vi "3DViewEye.vi"(0 "Choose Directory":path) -> ()   [LabVIEW 2022 SP3]
uses:
  <vilib>/Analysis/NI_AALPro.lvlib
  <vilib>/Analysis/4window.llb/Chebyshev Window (DBL).vi
  <vilib>/Math Plots/3D Math Plots/3D Surface/3D Surface Datatype/3D Surface Datatype.lvclass
  <vilib>/Math Plots/3D Math Plots/3D Surface/3D Surface Datatype/Public/Plot Helper (Vector).vi
  <vilib>/Math Plots/3D Math Plots/3D Surface/3D Surface XCtrl/3D Surface.xctl
panel:
  in  "length":i32
  in  "index":i32
  out "3D Surface":refnum<class "3D Plot Datatype.lvclass">[](xcontrol)
  out "Peaks":dbl[](graph)
  in  "# rings":i32=1
  in  "Fix dB Range?":bool
  in  "Parse":u16=1
  in  "Filter Prams":T1={"low cutoff"=5, "order"=81, "high cutoff"=35}
  in  "Type of Mean":u16(ring)=3 items=["Mean from lines", "Mean just lines", "Poly Mean", "No mean", "Filter"]
  in  "Flip?":bool=TRUE
  in  "Compress":bool
  in  "Y scale":dbl=1.0
  in  "X scale":dbl=1.0
  in  "file ext":string="*.eye"
  out "Current Image":string
  out "Numeric":i32
  out "Array":dbl[](array[numeric])
  in  "Save Data":bool
  in  "Use Selected Files":bool
  in  "Listbox":i32[](listbox)
  out "Scale factors":dbl[](array[numeric])
  out "BMP to be":dbl[][](graph)
  # "Slect a batch of eye files and the will be saved as BMP 24 bit RGB. They will be converted to a 1to1 aspect ratio and the batch will be scaled to reflect absolute voltage levels. Data is log compressed. May want to adjust Z scale to improve contrast."
  # "Scale in mm"
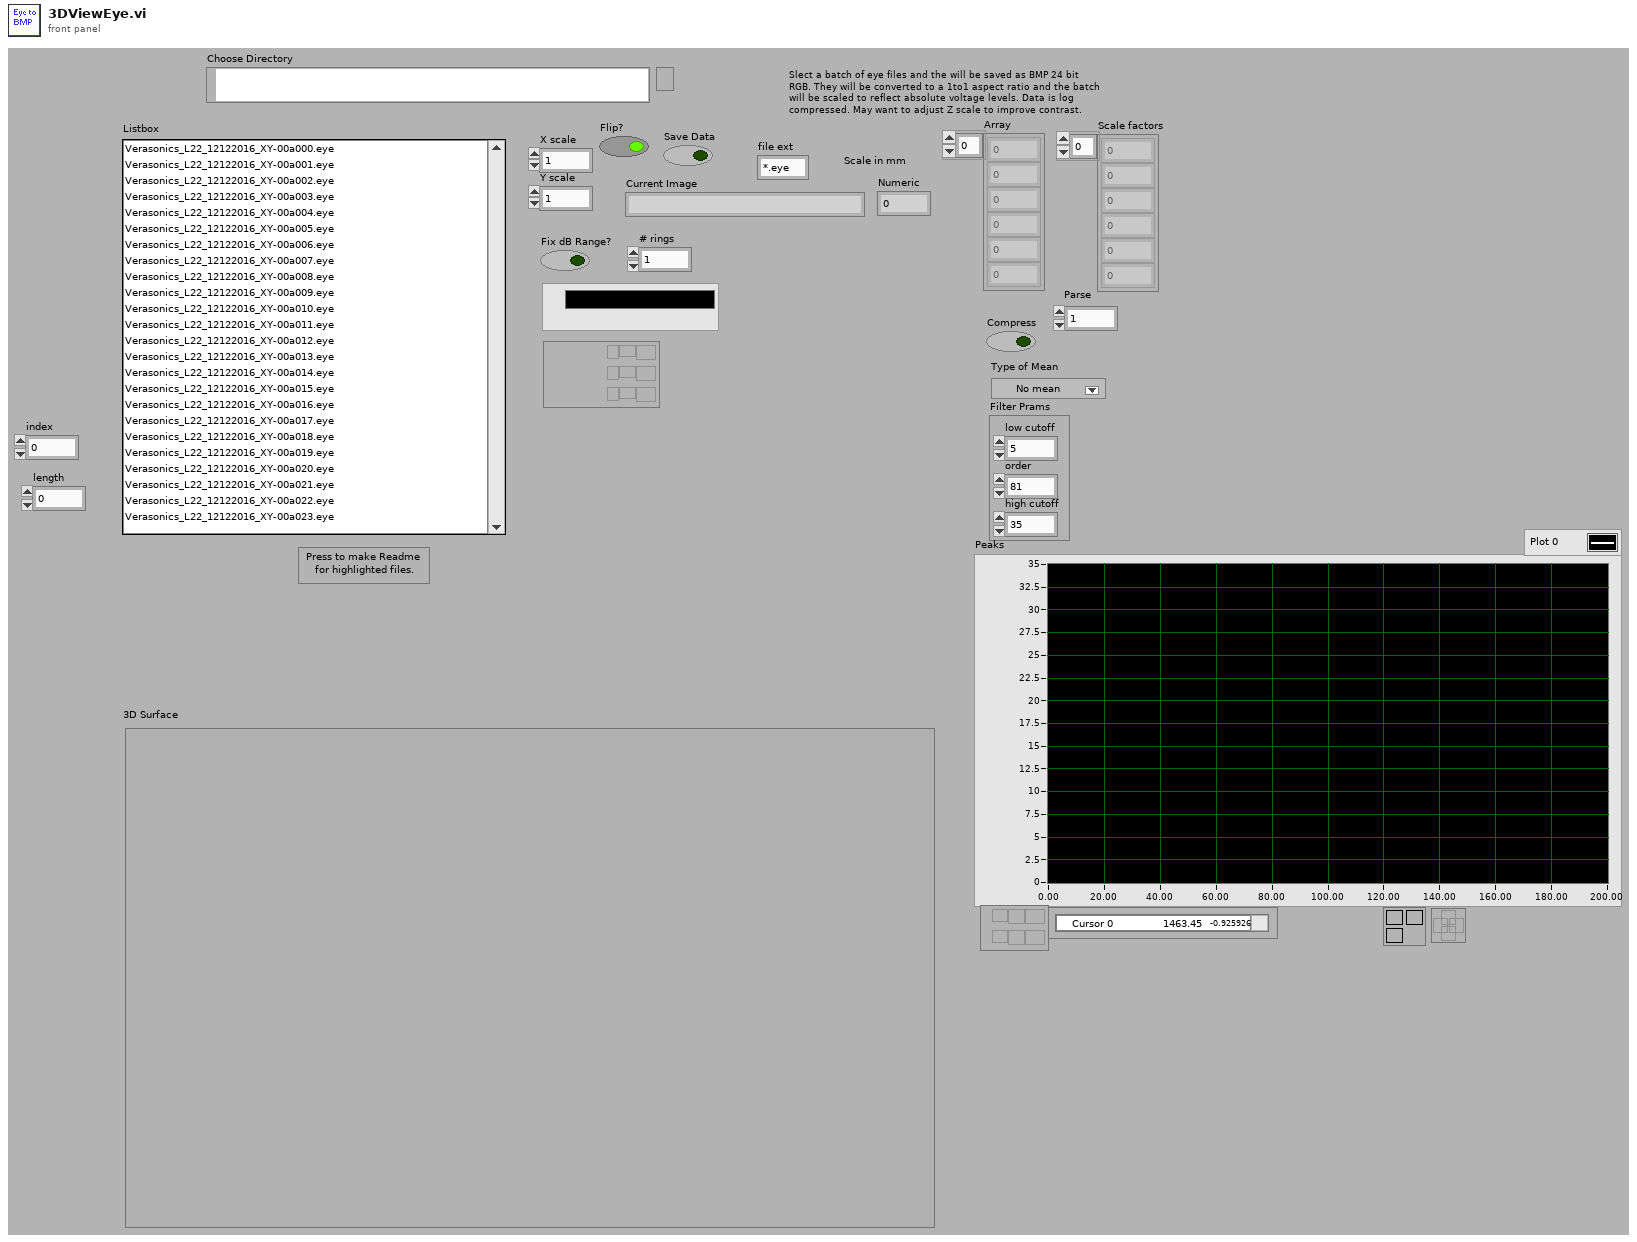
[diagram p1: front panel]
types:
  T1 = cluster{"low cutoff":i32, "order":i32, "high cutoff":i32}
  T2 = typedef "Header.ctl" = cluster{"header info":cluster{"Header":string, "Head length":i16}, "A/D info":cluster{"# rf points per line":u16, "# lines per scan":u16, "sample rate MHz":u16, "# A/D bits":i16, "# bytes per A/D":u16, "TGC Flag":u16, "A/D Type":string}, "Tranducer Info":cluster{"bandwidth":sgl, "center freq":sgl, "start freq":sgl, "ID":i32}, "Scan Info":cluster{"delay":sgl, "pivot distance":sgl, "sector scan angle":sgl, "operator":string, "Scan Mode":string, "location":string}, "Time/Date Info":cluster{"date":string, "time":string}, "RF Info":cluster{"RF file name":string, "RF file att":string, "RF cal file name":string, "RF cal file att":string}, "Patient Info":cluster{"ID":string, "extended ID":string, "age":u16, "sex":string, "previously\nscanned":string, "PSA":sgl, "LOS":u8, "Ethnicty 2":u8, "Race":u8}, "Tissue Type":cluster{"organ":i16, "disease type":i16, "disease location":i16, "IQ_pts":u16, "RcvBuffer":u8, "RcvFrame":u16, "IQBuff":u8, "IQFrame":u16, "IQPage":u8}, "Votage scaling":cluster{"Digitizer (dB)":sgl, "Gain (dB)":sgl, "Atten (dB)":sgl}, "Comment":string, "Misc Info":cluster{"avg num":u16, "c speed":i16, "Div By or SF zones":i16, "XMIT CHS":u8, "RCV CHS":u8, "Xmit angle":sgl}, "Therapy Parameters":cluster{"Theraputic Freq (MHz)":sgl, "Time on (s)":sgl, "Therapy amplitude (mV)":sgl, "Lines Before":u16, "Lines After":u16}, "Scan Settings":cluster{"Energy (uJ or V)":u8, "Damp (Ohm) or Fc":u8, "HP Filt (KHz)":u8, "LP Filt (MHz)":u8, "Gain (db)":u8, "prf (kHz)":sgl, "Distance between\nscan lines (um)":u16, "Distance between\nscan planes (um)":u16, "Scan line gap (um)":sgl, "Scan plane gap (um)":sgl}, "Compression Parameters":cluster{"F1 (MHz)":sgl, "F2 (MHz)":sgl, "% taper":sgl, "duration":sgl}, "Patient Info Xtra":cluster{"First Name":string, "Last Name":string, "Notes":string}, "ROI Box":u16[]}
  T3 = enum16{"None", "Stacked", "Clockwise", "Counterclockwise"}
  T4 = cluster{"F1 (MHz)":sgl, "F2 (MHz)":sgl, "% taper":sgl, "duration":sgl}
  T5 = cluster{cluster{dbl, dbl}, dbl, dbl, "delay":sgl, "delay":sgl, dbl, dbl}
  T6 = typedef "imagedata.ctl" = cluster{"image type":i32, "image depth":i32, "image":u8[], "mask":u8[], "colors":u32[], "Rectangle":cluster{"left":i16, "top":i16, "right":i16, "bottom":i16}}
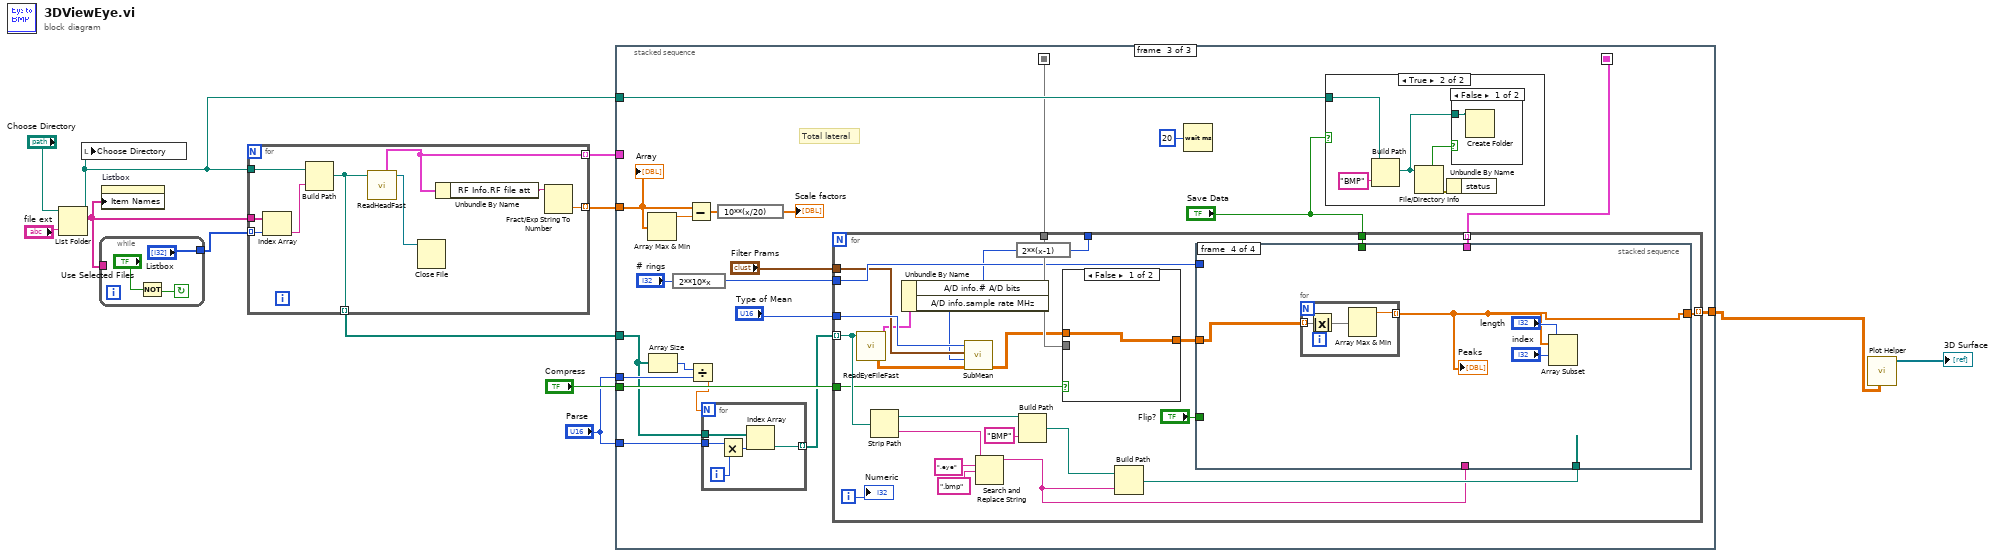
[diagram p0: block diagram]
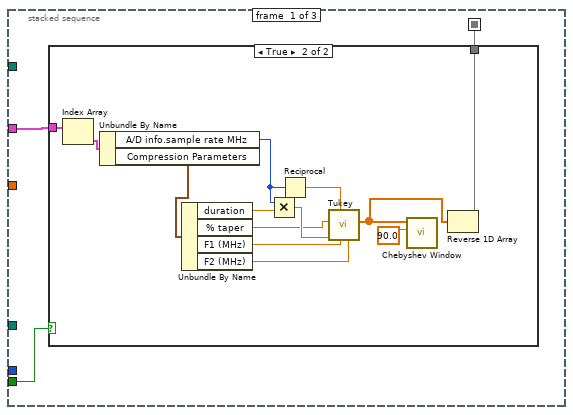
[diagram p2: hidden frame]
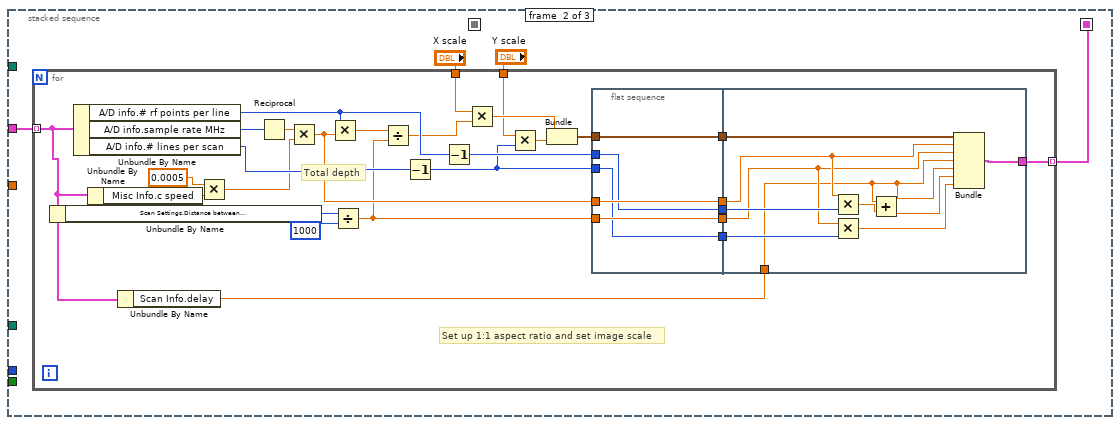
[diagram p4: hidden frame]
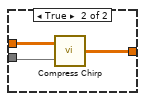
[diagram p7: hidden frame]
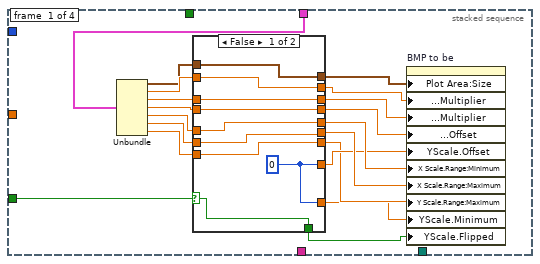
[diagram p8: hidden frame]
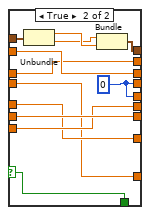
[diagram p9: hidden frame]
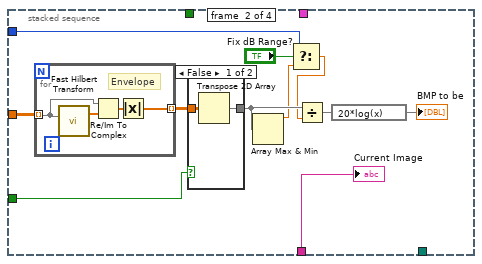
[diagram p10: hidden frame]
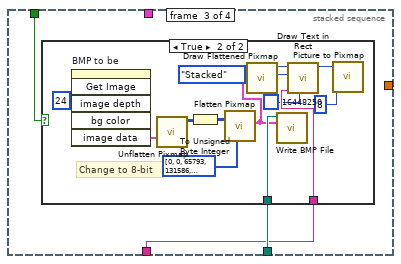
[diagram p12: hidden frame]
diagram:
  n1 = List Folder(path="Choose Directory", pattern="file ext") -> (path out=w6:path, filenames=w10:string[])  [unwired: 1 in, 3 out]
  n2 = local write "Choose Directory"(w6) -> ()
  n3 = while {
    tunnel: ["Listbox"] -> w9
    tunnel: w10 -> [_]
    stop <- w15 continue-if-true
    n4 = Not(x="Use Selected Files") -> (.not. x?=w15:bool)
  }
  n5 = property on="Listbox" class="LstBox (strict)"("Item Names"=w10) -> ()  [unwired: 2 in, 2 out]
  n6 = for {
    tunnel: [w23] -> w11 mode=indexing
    tunnel: [w17] -> w12 mode=indexing
    tunnel: w10 -> [w22]
    tunnel: w9 -> [w21] mode=indexing
    tunnel: [w18] -> w8 mode=indexing
    tunnel: w6 -> [w19]
    n7 = Index Array(array=w22, index=w21) -> (element=w20:string)
    n8 = Build Path(base path=w19, name or relative path=w20) -> (appended path=w18:path)
    n9 = call "ReadHeadFast.vi"("new file path"=w18) -> ("refnum out"=w16:refnum<file>, "Header In"=w17:T2)  [unwired: 7 in, 2 out]
    n10 = Close File(refnum=w16) -> ()  [unwired: 1 in, 2 out]
    n11 = Unbundle By Name(w17) -> ("RF Info.RF file att"=w24:string)
    n12 = Fract/Exp String To Number(string=w24) -> (number=w23:dbl)  [unwired: 4 out]
  }
  n13 = stacked-sequence {
    seq-local: [_ w43 _] -> [_ _ w102]
    seq-local: [w26 _ _] -> [_ _ w100]
    tunnel: w12 -> [w27 w44 _]
    tunnel: w11 -> [_ _ w108]
    tunnel: w8 -> [_ _ w93]
    tunnel: w6 -> [_ _ w105]
    tunnel: "Compress" -> [w25 _ w101]
    tunnel: "Parse" -> [_ _ w95]
    tunnel: "Parse" -> [_ _ w92]
    tunnel: [_ _ w88] -> w1
    frame #0 {
      n14 = case shown="True" w25 {
        tunnel: w27 -> [_ w32]
        tunnel: [_ w30] -> w26
        frame False {
        }
        frame True {
          n15 = Index Array(array=w32) -> (element=w31:T2)  [unwired: 1 in]
          n16 = Unbundle By Name(w31) -> ("A/D info.sample rate MHz"=w33:u16, "Compression Parameters"=w28:T4)
          n17 = Unbundle By Name(w28) -> ("duration"=w40:sgl, "% taper"=w35:sgl, "F1 (MHz)"=w39:sgl, "F2 (MHz)"=w38:sgl)
          n18 = Multiply(x=w33, y=w40) -> (x*y=w36:sgl)
          n19 = Reciprocal(x=w33) -> (1/x=w37:dbl)
          n20 = call "Tukey.vi"("f2 (MHz)"=w38, "f1 (MHz)"=w39, "Samp Rate (mics)"=w37, "Pts"=w36, "Tukey"=w35) -> ("Tukey Chirp"=w29:dbl[])  [unwired: 2 in, 4 out]
          n21 = call-poly <vilib>:"Chebyshev Window.vi"("lobe ratio (dB)"=90.0, "X"=w29) -> ()  [unwired: 10 out]
          n22 = Reverse 1D Array(array=w29) -> (reversed array=w30:dbl[])
        }
      }
    }
    frame #1 {
      n23 = for {
        tunnel: w44 -> [w45] mode=indexing
        tunnel: [w53] -> w43 mode=indexing
        tunnel: "X scale" -> [w47]
        tunnel: "Y scale" -> [w46]
        # "Set up 1:1 aspect ratio and set image scale"
        # "Total depth"
        n24 = Unbundle By Name(w45) -> ("Scan Settings.Distance between\nscan lines (um)"=w60:u16)
        n25 = Unbundle By Name(w45) -> ("A/D info.# rf points per line"=w63:u16, "A/D info.sample rate MHz"=w65:u16, "A/D info.# lines per scan"=w62:u16)
        n26 = Unbundle By Name(w45) -> ("Misc Info.c speed"=w59:i16)
        n27 = Unbundle By Name(w45) -> ("Scan Info.delay"=w55:sgl)
        n28 = Multiply(x=0.0005, y=w59) -> (x*y=w57:dbl)
        n29 = Reciprocal(x=w65) -> (1/x=w66:dbl)
        n30 = Multiply(x=w66, y=w57) -> (x*y=w56:dbl)
        n31 = Multiply(x=w63, y=w56) -> (x*y=w64:dbl)
        n32 = Divide(x=w60, y=1000) -> (x/y=w54:dbl)
        n33 = Divide(x=w64, y=w54) -> (x/y=w51:dbl)
        n34 = Decrement(x=w62) -> (x-1=w49:u16)
        n35 = Decrement(x=w63) -> (x-1=w61:u16)
        n36 = Multiply(x=w47, y=w51) -> (x*y=w50:dbl)
        n37 = Multiply(x=w46, y=w49) -> (x*y=w48:dbl)
        n38 = Bundle(w50, w48) -> (w52:cluster{dbl, dbl})  [unwired: 1 out]
        n39 = flat-sequence {
          tunnel: w61 -> [w74]
          tunnel: w49 -> [w75]
          tunnel: w52 -> [w73]
          tunnel: [w77] -> w72
          tunnel: w56 -> [w77]
          tunnel: [w76] -> w71
          tunnel: w54 -> [w76]
          tunnel: [w75] -> w70
          tunnel: [w74] -> w69
          tunnel: [w73] -> w68
          tunnel: w72 -> [w83]
          tunnel: w55 -> [w81]
          tunnel: w71 -> [w82]
          tunnel: w70 -> [w87]
          tunnel: w69 -> [w86]
          tunnel: w68 -> [w84]
          tunnel: [w78] -> w53
          frame #0 {
          }
          frame #1 {
            n40 = Multiply(x=w83, y=w86) -> (x*y=w85:dbl)
            n41 = Multiply(x=w82, y=w87) -> (x*y=w79:dbl)
            n42 = Add(x=w81, y=w85) -> (x+y=w80:dbl)
            n43 = Bundle(w84, w83, w82, "delay"=w81, "delay"=w81, w80, w79) -> (w78:T5)  [unwired: 1 out]
          }
        }
      }
    }
    frame #2 {
      # "Total lateral"
      n44 = Array Max & Min(array=w108) -> (max value=w107:dbl)  [unwired: 3 out]
      n45 = Array Size(array=w93) -> (size(s)=w96:i32)
      n46 = expression code="2**10*x"("# rings") -> (w98:i32)
      n47 = Subtract(x=w108, y=w107) -> (x-y=w104:dbl[])
      n48 = Divide(x=w96, y=w95) -> (x/y=w94:dbl)
      n49 = for {
        N: w94 -> [_]
        tunnel: w93 -> [w112]
        tunnel: w92 -> [w111]
        tunnel: [w110] -> w91 mode=indexing
        i -> [w113]
        n50 = Multiply(x=w111, y=w113) -> (x*y=w109:i32)
        n51 = Index Array(array=w112, index=w109) -> (element=w110:path)
      }
      n52 = expression code="10**(x/20)"(w104) -> (→"Scale factors":dbl[])
      n53 = for {
        tunnel: w91 -> [w145] mode=indexing
        tunnel: "Save Data" -> [w140]
        tunnel: w102 -> [w134] mode=indexing
        tunnel: "Type of Mean" -> [w133]
        tunnel: w101 -> [w132]
        tunnel: w100 -> [w131]
        tunnel: w98 -> [w126]
        tunnel: [w125] -> _
        tunnel: "Filter Prams" -> [w124]
        tunnel: [w120] -> w88 mode=indexing
        i -> [w139]
        n54 = call "ReadEyeFileFast.vi"("new file path"=w145) -> ("2-D data array"=w129:sgl[][], "Header In"=w123:T2)  [unwired: 1 in, 16 out]
        n55 = Strip Path(path=w145) -> (stripped path=w137:path, name=w144:string)
        n56 = Unbundle By Name(w123) -> ("A/D info.# A/D bits"=w121:i16, "A/D info.sample rate MHz"=w122:u16)
        n57 = call "SubMean.vi"("Scan Data In"=w129, "Samp Rate (MHz)"=w122, "Filter Prams"=w124, "Type of Mean"=w133) -> ("Array"=w130:dbl[][])  [unwired: 1 in, 2 out]
        n58 = Search and Replace String(input string=w144, search string=".eye", replace string=".bmp") -> (result string=w135:string)  [unwired: 1 in, 7 out]
        n59 = expression code="2**(x-1)"(w121) -> (w125:i16)
        n60 = Build Path(base path=w137, name or relative path="BMP") -> (appended path=w138:path)
        n61 = case shown="False" w132 {
          tunnel: w130 -> [w146 w149]
          tunnel: [w146 w148] -> w128
          tunnel: w131 -> [_ w147]
          frame False {
          }
          frame True {
            n62 = call "Compress Chirp.vi"("Chirp"=w147, "Array In"=w149) -> ("Array Out"=w148:dbl[][])
          }
        }
        n63 = Build Path(base path=w138, name or relative path=w135) -> (appended path=w141:path)
        n64 = stacked-sequence {
          tunnel: w135 -> [_ w200 w208 _]
          tunnel: w141 -> [_ _ w210 _]
          tunnel: w140 -> [_ _ w209 _]
          tunnel: w134 -> [w168 _ _ _]
          tunnel: w128 -> [_ w198 _ w227]
          tunnel: "Flip?" -> [w152 w196 _ _]
          tunnel: w126 -> [_ w193 _ _]
          tunnel: [_ _ _ w224] -> w120
          frame #0 {
            n65 = Unbundle(w168) -> (w161:cluster{dbl, dbl}, w162:dbl, w167:dbl, "delay"=w166:sgl, "delay"=w165:sgl, w164:dbl, w163:dbl)
            n66 = case shown="False" w152 {
              selector: w152 -> [w169 w178]
              tunnel: [w177 w189] -> w158
              tunnel: w167 -> [w177 w188]
              tunnel: [w176 w180] -> w157
              tunnel: w166 -> [w176 w179]
              tunnel: [w170 w180] -> w156
              tunnel: w165 -> [w170 w181]
              tunnel: [w172 w186] -> w155
              tunnel: w164 -> [w172 w187]
              tunnel: [w175 w187] -> w153
              tunnel: w163 -> [w175 w186]
              tunnel: [w174 w188] -> w159
              tunnel: w162 -> [w174 w189]
              tunnel: [w173 w182] -> w160
              tunnel: w161 -> [w173 w185]
              tunnel: [w171 w181] -> w154
              tunnel: [w171 w179] -> w151
              tunnel: [w169 w178] -> w150
              frame False {
                w171 = 0
              }
              frame True {
                w180 = 0
                n67 = Unbundle(w185) -> (w184:dbl, w183:dbl)
                n68 = Bundle(w183, w184) -> (w182:cluster{dbl, dbl})  [unwired: 1 in]
              }
            }
            n69 = property on="BMP to be" class="IntGraph (strict)"("Plot Area:Size"=w160, "X Scale.Offset and Multiplier:Multiplier"=w159, "Y Scale.Offset and Multiplier:Multiplier"=w158, "X Scale.Offset and Multiplier:Offset"=w157, "YScale.Offset"=w154, "X Scale.Range:Minimum"=w156, "X Scale.Range:Maximum"=w155, "Y Scale.Range:Maximum"=w153, "YScale.Minimum"=w151, "YScale.Flipped"=w150) -> ()  [unwired: 2 in, 2 out]
          }
          frame #1 {
            n70 = for {
              tunnel: w198 -> [w204] mode=indexing
              tunnel: [w205] -> w197 mode=indexing
              # "Envelope"
              n71 = call <vilib>:"Fast Hilbert Transform.vi"("X"=w204) -> ("Hilbert{X}"=w206:dbl[])  [unwired: 1 out]
              n72 = Re/Im To Complex(1:w206, 2:w204) -> (0:w207:cdb[])
              n73 = Absolute Value(x=w207) -> (abs(x)=w205:dbl[])
            }
            n74 = case shown="False" w196 {
              tunnel: w197 -> [w202 w203]
              tunnel: [w201 w203] -> w195
              frame False {
                n75 = Transpose 2D Array(2D array=w202) -> (transposed array=w201:dbl[][])
              }
              frame True {
              }
            }
            n76 = Array Max & Min(array=w195) -> (max value=w192:dbl)  [unwired: 3 out]
            n77 = Select(t=w193, s="Fix dB Range?", f=w192) -> (s? t:f=w191:dbl)
            n78 = Divide(x=w195, y=w191) -> (x/y=w194:dbl[][])
            n79 = expression code="20*log(x)"(w194) -> (→"BMP to be":dbl[][])
            "Current Image" <- w200
          }
          frame #2 {
            n80 = case shown="True" w209 {
              tunnel: w210 -> [_ w221]
              tunnel: w208 -> [_ w216]
              frame False {
              }
              frame True {
                # "Change to 8-bit"
                n81 = invoke on="BMP to be" class="IntGraph (strict)" method="Get Image"("image depth"=24) -> ("image data"=w222:T6)  [unwired: 5 in, 5 out]
                n82 = call <vilib>:"Unflatten Pixmap.vi"("image data"=w222) -> ("24-bit pixmap"=w219:u32[][])  [unwired: 10 out]
                n83 = To Unsigned Byte Integer(number=w219) -> (unsigned 8bit integer=w218:u8[][])
                n84 = call <vilib>:"Flatten Pixmap.vi"("colors"=u32[] [0, 0, 65793, 131586, 197379, 263172, 328965, 394758, 460551, 526344, 592137, 657930, 723723, 789516, 855309, 921102, 986895, 1052688, 1118481, 1184274, 1250067, 1315860, 1381653, 1447446, 1513239, 1579032, 1644825, 1710618, 1776411, 1842204, 1907997, 1973790, 2039583, 2105376, 2171169, 2236962, 2302755, 2368548, 2434341, 2500134, 2565927, 2631720, 2697513, 2763306, 2829099, 2894892, 2960685, 3026478, 3092271, 3158064, 3223857, 3289650, 3355443, 3421236, 3487029, 3552822, 3618615, 3684408, 3750201, 3815994, 3881787, 3947580, 4013373, 4079166, 4144959, 4210752, 4276545, 4342338, 4408131, 4473924, 4539717, 4605510, 4671303, 4737096, 4802889, 4868682, 4934475, 5000268, 5066061, 5131854, 5197647, 5263440, 5329233, 5395026, 5460819, 5526612, 5592405, 5658198, 5723991, 5789784, 5855577, 5921370, 5987163, 6052956, 6118749, 6184542, 6250335, 6316128, 6381921, 6447714, 6513507, 6579300, 6645093, 6710886, 6776679, 6842472, 6908265, 6974058, 7039851, 7105644, 7171437, 7237230, 7303023, 7368816, 7434609, 7500402, 7566195, 7631988, 7697781, 7763574, 7829367, 7895160, 7960953, 8026746, 8092539, 8158332, 8224125, 8289918, 8355711, 8421504, 8487297, 8553090, 8618883, 8684676, 8750469, 8816262, 8882055, 8947848, 9013641, 9079434, 9145227, 9211020, 9276813, 9342606, 9408399, 9474192, 9539985, 9605778, 9671571, 9737364, 9803157, 9868950, 9934743, 10000536, 10066329, 10132122, 10197915, 10263708, 10329501, 10395294, 10461087, 10526880, 10592673, 10658466, 10724259, 10790052, 10855845, 10921638, 10987431, 11053224, 11119017, 11184810, 11250603, 11316396, 11382189, 11447982, 11513775, 11579568, 11645361, 11711154, 11776947, 11842740, 11908533, 11974326, 12040119, 12105912, 12171705, 12237498, 12303291, 12369084, 12434877, 12500670, 12566463, 12632256, 12698049, 12763842, 12829635, 12895428, 12961221, 13027014, 13092807, 13158600, 13224393, 13290186, 13355979, 13421772, 13487565, 13553358, 13619151, 13684944, 13750737, 13816530, 13882323, 13948116, 14013909, 14079702, 14145495, 14211288, 14277081, 14342874, 14408667, 14474460, 14540253, 14606046, 14671839, 14737632, 14803425, 14869218, 14935011, 15000804, 15066597, 15132390, 15198183, 15263976, 15329769, 15395562, 15461355, 15527148, 15592941, 15658734, 15724527, 15790320, 15856113, 15921906, 15987699, 16053492, 16119285, 16185078, 16250871, 16316664, 16382457, 16448250, 16514043, 16579836, 16645629, 16448250] ("Array 2"), "8-bit pixmap"=w218) -> ("image data"=w211:T6)  [unwired: 4 in, 5 out]
                n85 = call <vilib>:"Draw Flattened Pixmap.vi"("image data"=w211) -> ("new picture"=w217:picture)  [unwired: 8 in]
                n86 = call <vilib>:"Write BMP File.vi"("image data"=w211, "path to BMP file"=w221) -> ()  [unwired: 1 in, 9 out]
                n87 = call <vilib>:"Draw Text in Rect.vi"("text color(black)"=u32 16448250, "text"=w216, "text orientation"=T3."Stacked", "picture"=w217) -> ("new picture"=w215:picture)  [unwired: 7 in]
                n88 = call <vilib>:"Picture to Pixmap.vi"("depth"=8, "picture"=w215) -> ()  [unwired: 8 in, 2 out]
              }
            }
          }
          frame #3 {
            n89 = for {
              tunnel: [w230] -> w224 mode=indexing
              tunnel: w227 -> [w229] mode=indexing
              n90 = Absolute Value(x=w229) -> (abs(x)=w228:dbl[])
              n91 = Array Max & Min(array=w228) -> (max value=w230:dbl)  [unwired: 3 out]
            }
            "Peaks" <- w224
            n92 = Array Subset(array=w224, index="index", length="length") -> ()  [unwired: 1 out]
          }
        }
        "Numeric" <- w139
      }
      n93 = Wait (ms)(milliseconds to wait=u32 20) -> ()  [unwired: 1 out]
      n94 = case shown="True" "Save Data" {
        tunnel: w105 -> [_ w114]
        frame False {
        }
        frame True {
          n95 = Build Path(base path=w114, name or relative path="BMP") -> (appended path=w116:path)
          n96 = File/Directory Info(path=w116) -> (directory=w115:bool, error out=w117:errorcluster)  [unwired: 1 in, 5 out]
          n97 = Unbundle By Name(w117) -> ()  [unwired: 1 out]
          n98 = case shown="False" w115 {
            tunnel: w116 -> [w119 _]
            frame False {
              n99 = Create Folder(path (use dialog)=w119) -> ()  [unwired: 1 in, 4 out]
            }
            frame True {
            }
          }
        }
      }
      "Array" <- w108
    }
  }
  n100 = call-poly <vilib>:"Plot Helper.vi"("z matrix"=w1) -> ("3D Plot lvclass Array out"=→"3D Surface":refnum<class "3D Plot Datatype.lvclass">[])  [unwired: 5 in, 5 out]
